vi "Save Recall Setup.vi"(8 "error in (no error)":errorcluster, 9 "Memory Setup (1)":i32=1 min=1 max=20 step=1, 10 "Operation Mode (0:Save)":i32(ring) items=["Save", "Recall"], 11 "VISA resource name":refnum<visa-resource-name>) -> (0 "error out":errorcluster, 3 "VISA resource name out":refnum<visa-resource-name>)   [LabVIEW 2015, in "Siglent SPD3000 Series.lvlib"]
doc: "Stores or recalls the current state of your instrument in/from non-volatile internal memory. Stores the complete front panel setup of the oscilloscope at the time the command is issued, or setup front panel from non-volatile internal memory."
uses:
  <instrlib>/Siglent SPD3000 Series/Siglent SPD3000 Series.lvlib
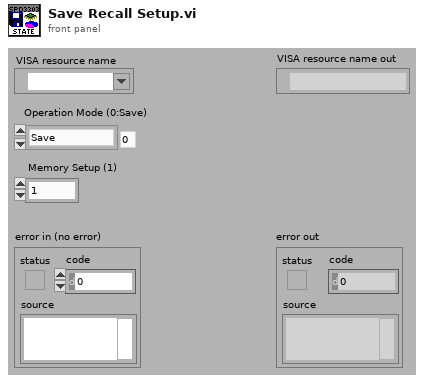
[diagram p1: front panel]
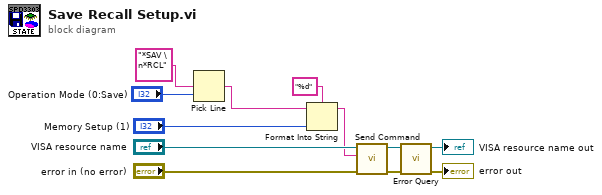
[diagram p0: block diagram]
diagram:
  n1 = Pick Line(multi-line string="*SAV \n*RCL", line index="Operation Mode (0:Save)") -> (output string=w3:string)  [unwired: 1 in]
  n2 = Format Into String(format string="%d", initial string=w3, "Memory Setup (1)") -> (resulting string=w4:string)  [unwired: 1 in, 1 out]
  n3 = call <instrlib>:"Send Command.vi"("error in (no error)"="error in (no error)", "Write Buffer (\"\")"=w4, "VISA resource name"="VISA resource name") -> ("error out"=w7:errorcluster, "VISA resource name out"=w8:refnum<visa-resource-name>)  [unwired: 7 in]
  n4 = call <instrlib>:"Error Query.vi"("error in (no error)"=w7, "VISA resource name"=w8) -> ("error out"=→"error out":errorcluster, "VISA resource name out"=→"VISA resource name out":refnum<visa-resource-name>)  [unwired: 6 in, 2 out]
